vi "TrigPulse.vi"(1 "error in":errorcluster, 2 "Generator ID":T1 caption="RIO Device") -> (0 "error out":errorcluster)   [LabVIEW 2018]
uses:
  <vilib>/userdefined/High Color/nirio_resource_hc.ctl
  <vilib>/Utility/error.llb/Error Cluster From Error Code.vi
  <vilib>/rvi/errors/niLvFpgaAdjustHostInterfaceError.vi
  <vilib>/FPGAPlugInAG/Dynamic/niLvFpga_Close_Dynamic.vi
  <vilib>/rvi/interface/nirviReadWriteControl/nirviReadWriteControl.xnode
  <vilib>/rvi/interface/nirviCloseFPGA/nirviCloseFPGA.xnode
  NiFpgaLv.dll
  <vilib>/rvi/interface/Simulation/niFpgaSimulationCallBeginRW.vi
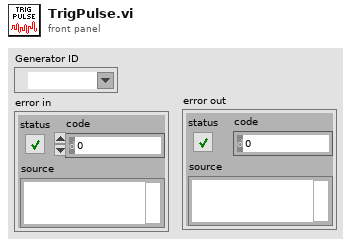
[diagram p1: front panel]
types:
  T1 = typedef "nirio_resource_hc.ctl" = tag
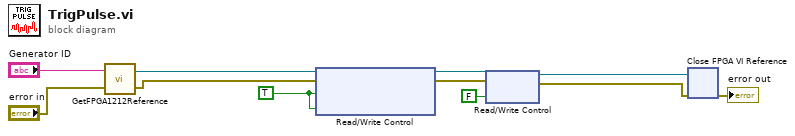
[diagram p0: block diagram]
diagram:
  w5 = TRUE ("Trig In")
  n1 = call "GetFPGA1212Reference.vi"("error in"="error in", "RIO Device IN"="Generator ID") -> ("error out"=w3:errorcluster, "FPGA VI Reference Out"=w2:refnum<k20>)
  n2 = xnode "Read/Write Control"("FPGA VI Reference In"=w2, "error in"=w3, "Trig In"=w5, "Vi_Trig/nStage_Trig"=w5) -> ("FPGA VI Reference Out"=w11:refnum<k20>, "error out"=w10:errorcluster)
  n3 = xnode "Read/Write Control"("FPGA VI Reference In"=w11, "error in"=w10, "Trig In"=FALSE) -> ("FPGA VI Reference Out"=w9:refnum<k20>, "error out"=w8:errorcluster)
  n4 = xnode "Close FPGA VI Reference"("FPGA VI Reference In"=w9, "error in"=w8) -> ("error out"=→"error out":errorcluster)
